vi "Move Z.vi"(0 "ASI stage":T1, 9 "z":dbl, 11 "error in (no error)":errorcluster) -> (15 "error out":errorcluster)   [LabVIEW 2010]
uses:
  stage properties.ctl
panel:
  in  "y":dbl
  in  "x":dbl
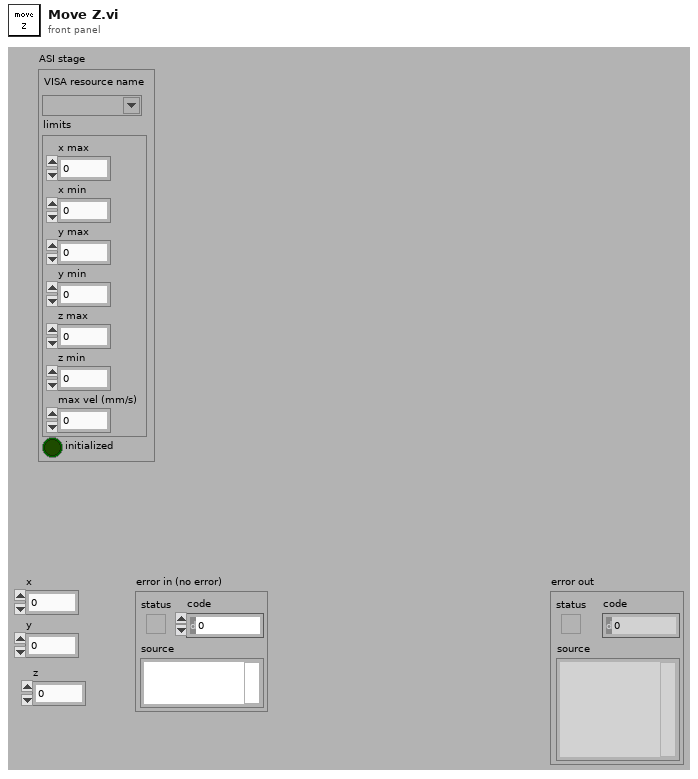
[diagram p1: front panel]
types:
  T1 = typedef "stage properties.ctl" = cluster{"VISA resource name":refnum<visa-resource-name>, "limits":cluster{"x max":dbl, "x min":dbl, "y max":dbl, "y min":dbl, "z max":dbl, "z min":dbl, "max vel (mm/s)":dbl}, "initialized":bool}
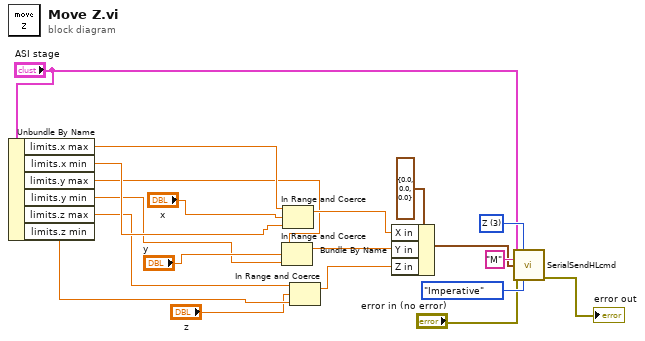
[diagram p0: block diagram]
diagram:
  w20 = u16 3 items=["No axis", "X", "Y", "Z", "XY", "XYZ"] ("Axis configuration")
  n1 = Unbundle By Name("ASI stage") -> ("limits.x max"=w15:dbl, "limits.x min"=w8:dbl, "limits.y max"=w7:dbl, "limits.y min"=w6:dbl, "limits.z max"=w5:dbl, "limits.z min"=w4:dbl)
  n2 = In Range and Coerce(upper limit=w7, x="y", lower limit=w6) -> (coerced(x)=w12:dbl)  [unwired: 1 out]
  n3 = In Range and Coerce(upper limit=w15, x="x", lower limit=w8) -> (coerced(x)=w11:dbl)  [unwired: 1 out]
  n4 = In Range and Coerce(upper limit=w5, x="z", lower limit=w4) -> (coerced(x)=w2:dbl)  [unwired: 1 out]
  n5 = Bundle By Name(cluster=cluster{"X in":dbl, "Y in":dbl, "Z in":dbl} {"X in"=0.0, "Y in"=0.0, "Z in"=0.0} ("data in"), "X in"=w11, "Y in"=w12, "Z in"=w2) -> (w10:cluster{"X in":dbl, "Y in":dbl, "Z in":dbl})
  n6 = call "SerialSendHLcmd.vi"("ASI stage"="ASI stage", "Axis configuration"=w20, "Command"="M", "data in"=w10, "error in (no error)"="error in (no error)", "Command type"=enum16{"Query", "Where", "Imperative", "DU Y"}."Imperative") -> ("error out"=→"error out":errorcluster)  [unwired: 7 in, 2 out]
